vi "WhileLoop.vi"(8 "error in":errorcluster, 11 "reference":refnum<vi>) -> (0 "error out":errorcluster, 3 "WhileLoop out":refnum<class "WhileLoop.lvclass">)   [LabVIEW 2014, in "WhileLoop.lvclass"]
uses:
  WhileLoop.lvclass
  WhileLoop.lvclass/WhileLoop.ctl
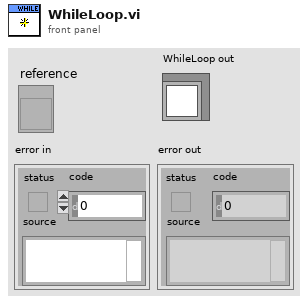
[diagram p1: front panel]
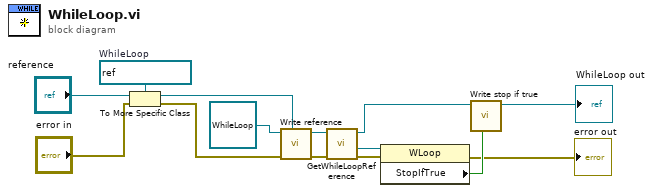
[diagram p0: block diagram]
diagram:
  w13 = refnum<vi> refnum  # WhileLoop
  n1 = To More Specific Class(target class=w13, reference="reference", error in="error in") -> (specific class reference=w10:refnum<vi>, error out=w11:errorcluster)
  n2 = call-dynamic "Write reference.vi"("reference"=w10, "error in"=w11, "GObject in"=refnum<class "WhileLoop.lvclass"> refnum ("ForLoop in")) -> ("error out"=w8:errorcluster, "GObject out"=w9:refnum<class "WhileLoop.lvclass">)  [unwired: 5 in]
  n3 = call "GetWhileLoopReference.vi"("error in"=w8, "WhileLoop in"=w9) -> ("error out"=w5:errorcluster, "reference out"=w7:refnum<vi>, "WhileLoop out"=w4:refnum<class "WhileLoop.lvclass">)  [unwired: 7 in]
  n4 = property class="WLoop"(reference=w7, error in=w5) -> (error out=→"error out":errorcluster, "StopIfTrue"=w3:bool)  [unwired: 1 out]
  n5 = call "Write stop if true.vi"("stop if true"=w3, "ForLoop in"=w4) -> ("ForLoop out"=→"WhileLoop out":refnum<class "WhileLoop.lvclass">)  [unwired: 7 in]
